vi "Beak Controller.vi"(8 "error in":errorcluster) -> ()   [LabVIEW 2018]
doc: "This VI executes continuously carrying out the current operation and responding to updates or new operations. It will often contain the timing or control code that is difficult to place directly in TeleOp. This VI generally opens all sensors and motors and isolates the rest of the robot code from knowing how the operations are carried out."
uses:
  <vilib>/Rock Robotics/WPI/Framework/Completion Status.ctl
  Beak Setpoints.ctl
  Beak Operations.ctl
  <vilib>/Rock Robotics/WPI/Solenoid/WPI_SolenoidValue.ctl
  <vilib>/Rock Robotics/WPI/Solenoid/WPI_SolenoidDevRef.ctl
  <vilib>/Rock Robotics/WPI/Solenoid/WPI_SolenoidChannel.ctl
  <vilib>/Rock Robotics/WPI/Counter/WPI_CounterDevRef.ctl
  <vilib>/Rock Robotics/SystemInterfaces/Counter/FPGA_CounterCtrSystemIndex.ctl
  <vilib>/Rock Robotics/WPI/Solenoid/WPI_SolenoidSetEnum.vi
  Beak Published Globals.vi
  Wrist/Implementation/Wrist Published Globals.vi
panel:
  in  "Wrist Block Angle":dbl=80.0
  in  "Sensor Distance mm":dbl=60.0
  out "Waveform Chart":dbl(graph)
  out "Distance mm":dbl
  in  "Extend Polarity":T1=enum."Reverse"
  in  "Open Polarity":T1=enum."Reverse"
  in  "Interactive Values":T2
  out "Current\nCmd":string
  in  "Buttons":cluster{"Execute Cmd":bool, "Abort Cmd":bool}
  out "Command Timing":cluster{"Start Time (ms)":u32, "Iterations":i32}
  out "Status":T4
  # "Interactive Command: You may fill in the settings for a command\nand schedule it with the Execute button. You can observe and abort\nany command while fine tuning the code for the controller."
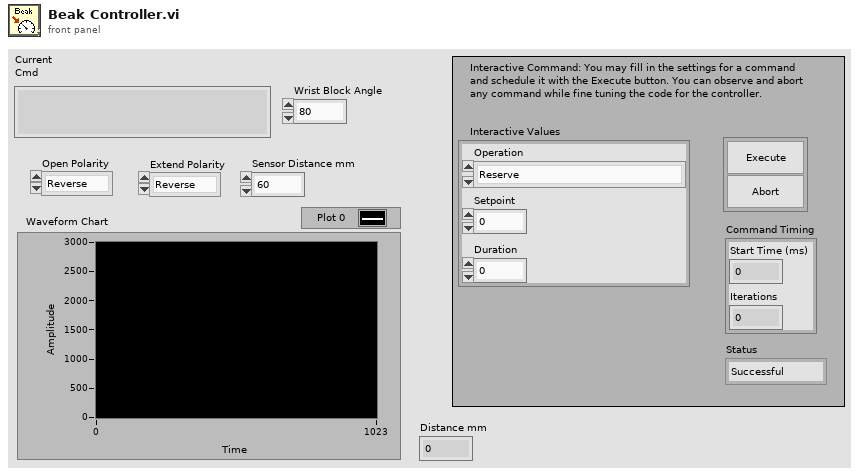
[diagram p1: front panel]
types:
  T1 = typedef "WPI_SolenoidValue.ctl" = enum16{"Off", "On", "Forward", "Reverse"}
  T2 = typedef "Beak Setpoints.ctl" = cluster{"Operation":T3, "Setpoint":dbl, "Duration":dbl}
  T3 = typedef "Beak Operations.ctl" = enum16{"Reserve", "Read Current", "Immediate", "Open", "Close", "Extend", "Retract"}
  T4 = typedef "Completion Status.ctl" = enum16{"Successful", "Aborted", "Incomplete"}
  T5 = typedef "WPI_SolenoidDevRef.ctl" = cluster{"DevStatus":errorcluster, "Pneumatics Control Module":u8, "Forward Solenoid Channel":T6, "Reverse Solenoid Channel":T6}
  T6 = typedef "WPI_SolenoidChannel.ctl" = enum8{"Solenoid 0", "Solenoid 1", "Solenoid 2", "Solenoid 3", "Solenoid 4", "Solenoid 5", "Solenoid 6", "Solenoid 7", "Invalid"}
  T7 = typedef "WPI_CounterDevRef.ctl" = cluster{"DevStatus":errorcluster, "CntIndex":T8}
  T8 = typedef "FPGA_CounterCtrSystemIndex.ctl" = enum8{"Ctr 0", "Ctr 1", "Ctr 2", "Ctr 3", "Ctr 4", "Ctr 5", "Ctr 6", "Ctr 7", "Invalid"}
  T9 = cluster{"Beak":T5, "BeakExtension":T5, "Hatch Sensor":T7}
  T10 = typedef "Command Status Info.ctl" = cluster{"Name":string, "Status":T4, "notifier out":T11}
  T11 = typedef "Completion Notifier.ctl" = refnum<notifier>
  T12 = cluster{"Current Command":T2, "Command Timing":cluster{"Start Time (ms)":u32, "Iterations":i32}, "Command Arguments":cluster{"Command Info":T10, "Description":string, "Default Command":T2, "queue out":refnum<queue>, "Subsystem Name":string}}
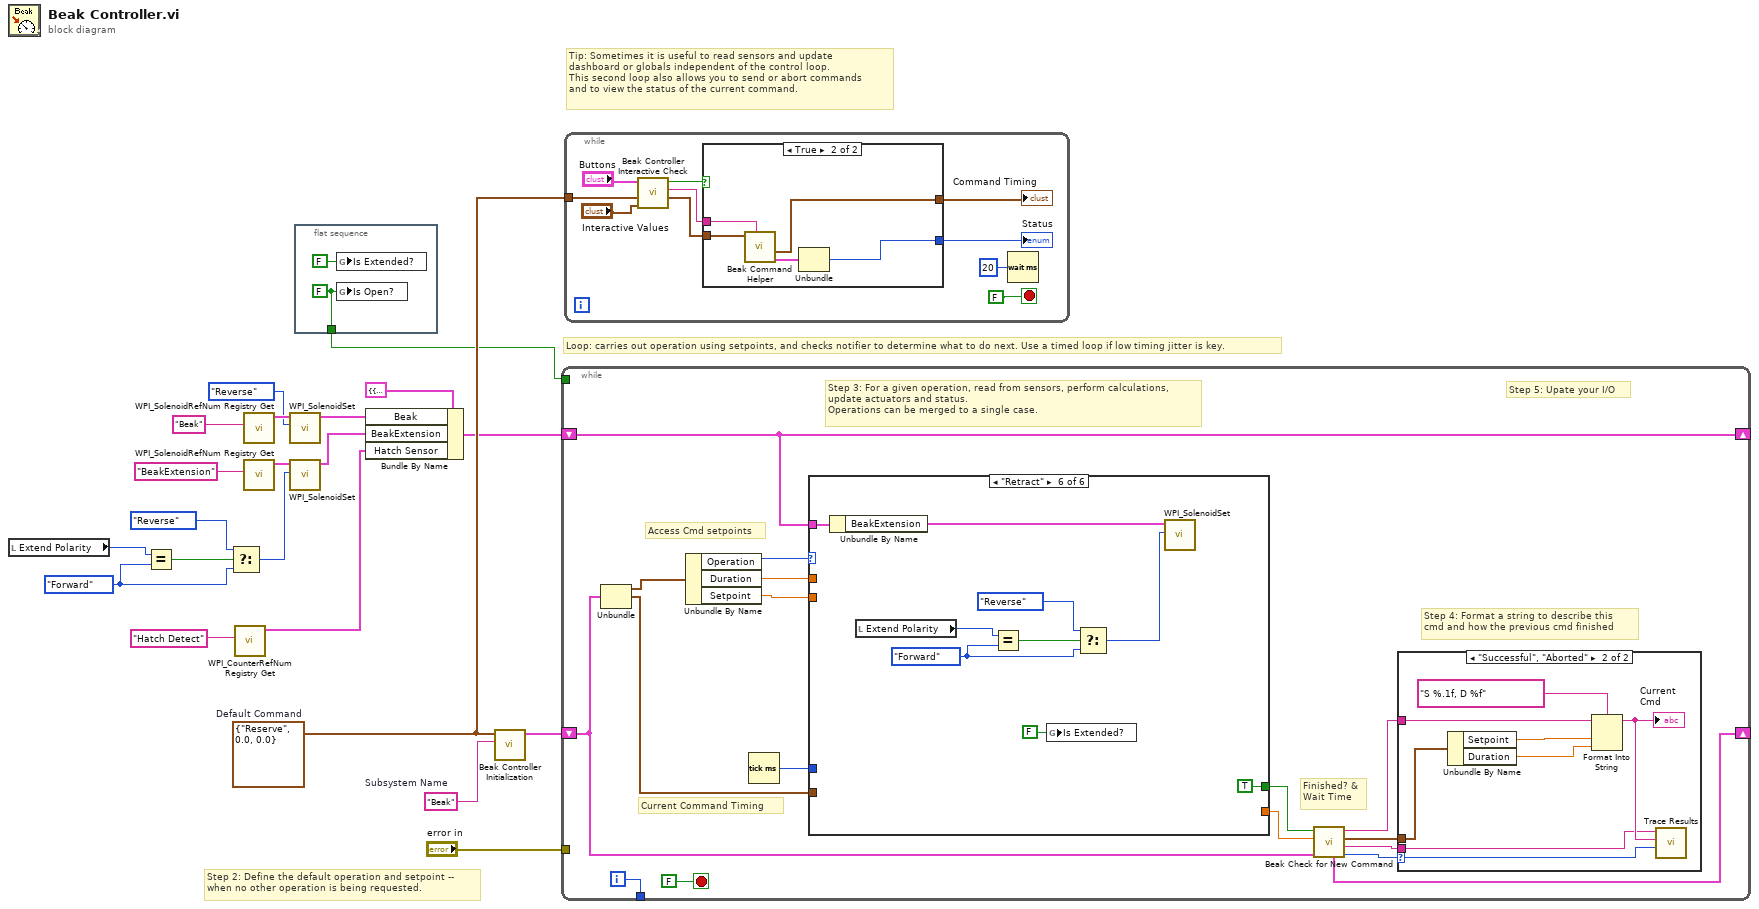
[diagram p0: block diagram]
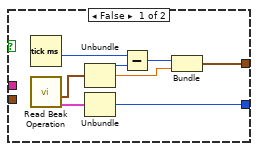
[diagram p2: hidden frame]
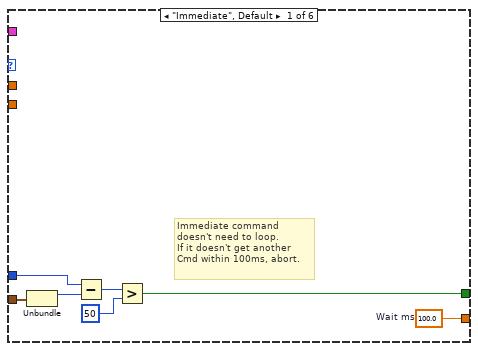
[diagram p4: hidden frame]
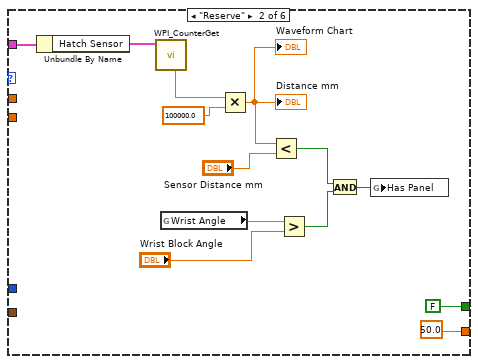
[diagram p5: hidden frame]
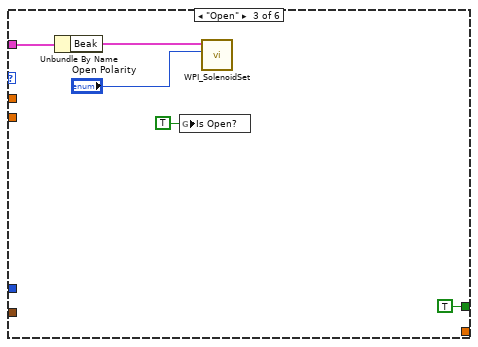
[diagram p6: hidden frame]
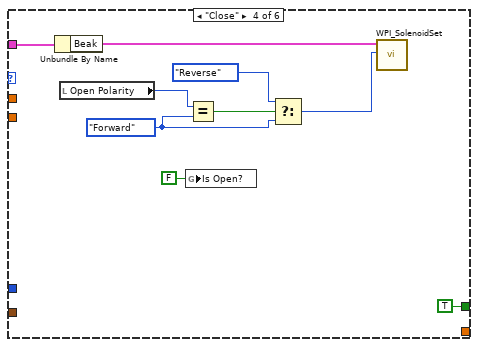
[diagram p7: hidden frame]
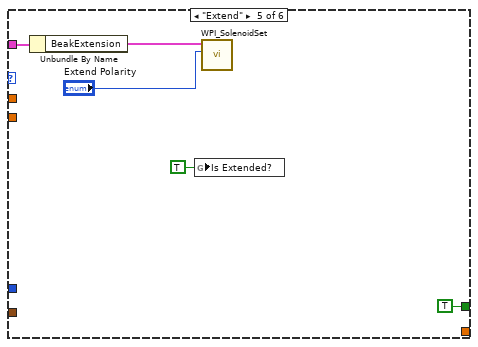
[diagram p8: hidden frame]
diagram:
  w9 = WPI_SolenoidValue."Forward" ("y")
  w18 = T2 {"Operation"=enum."Reserve", "Setpoint"=0.0, "Duration"=0.0}  # Default Command
  w19 = "Beak"  # Subsystem Name
  # "Tip: Sometimes it is useful to read sensors and update\ndashboard or globals independent of the control loop.\nThis second loop also allows you to send or abort commands\nand to view the status of the current command."
  # "Step 2: Define the default operation and setpoint --\nwhen no other operation is being requested."
  # "Loop: carries out operation using setpoints, and checks notifier to determine what to do next. Use a timed loop if low timing jitter is key."
  n1 = local read "Extend Polarity"() -> (w6:T1)
  n2 = Equal?(x=w6, y=w9) -> (x = y?=w7:bool)
  n3 = Select(t=WPI_SolenoidValue."Reverse" ("y"), s=w7, f=w9) -> (s? t:f=w5:T1)
  n4 = call <vilib>:"WPI_CounterRefNum Registry Get.vi"("refnum name"="Hatch Detect") -> ("CounterDevRef"=w3:T7)  [unwired: 9 in, 1 out]
  n5 = call <vilib>:"WPI_SolenoidRefNum Registry Get.vi"("refnum name"="Beak") -> ("SolenoidDevRef"=w13:T5)  [unwired: 9 in, 1 out]
  n6 = call <vilib>:"WPI_SolenoidRefNum Registry Get.vi"("refnum name"="BeakExtension") -> ("SolenoidDevRef"=w11:T5)  [unwired: 9 in, 1 out]
  n7 = call-poly <vilib>:"WPI_SolenoidSet.vi"("Value"=WPI_SolenoidValue."Reverse" ("y"), "SolenoidDevRef"=w13) -> ("SolenoidDevRef"=w12:T5)  [unwired: 8 in, 1 out]
  n8 = call-poly <vilib>:"WPI_SolenoidSet.vi"("Value"=w5, "SolenoidDevRef"=w11) -> ("SolenoidDevRef"=w10:T5)  [unwired: 8 in, 1 out]
  n9 = flat-sequence {
    tunnel: [w22] -> w2
    frame #0 {
      w22 = FALSE ("Is Open?")
      n10 = global write "Beak Published Globals.vi" "Is Extended?"(FALSE ("Is Extended?")) -> ()
      n11 = global write "Beak Published Globals.vi" "Is Open?"(w22) -> ()
    }
  }
  n12 = Bundle By Name(cluster=T9 {"Beak"={"DevStatus"={"status"=FALSE, "code"=0, "source"=""}, "Pneumatics Control Module"=0, "Forward Solenoid Channel"=enum."Invalid", "Reverse Solenoid Channel"=enum."Invalid"}, "BeakExtension"={"DevStatus"={"status"=FALSE, "code"=0, "source"=""}, "Pneumatics Control Module"=0, "Forward Solenoid Channel"=enum."Invalid", "Reverse Solenoid Channel"=enum."Invalid"}, "Hatch Sensor"={"DevStatus"={"status"=FALSE, "code"=0, "source"=""}, "CntIndex"=enum."Ctr 0"}}, "Beak"=w12, "BeakExtension"=w10, "Hatch Sensor"=w3) -> (w14:T9)
  n13 = call "Beak Controller Initialization.vi"("Subsystem Name"=w19, "Default Command"=w18) -> ("Current Command"=w20:T12)  [unwired: 9 in]
  n14 = while {
    shift-right: [w32] -> _
    shift-left: w20 -> [w25]
    tunnel: [w39] -> _
    tunnel: "error in" -> [_]
    shift-right: [w24] -> _
    shift-left: w14 -> [w24]
    tunnel: w2 -> [_]
    i -> [w39]
    stop <- FALSE stop-if-true
    # "Step 5: Upate your I/O"
    # "Step 4: Format a string to describe this\ncmd and how the previous cmd finished"
    # "Current Command Timing"
    # "Access Cmd setpoints"
    # "Finished? &\nWait Time"
    # "Step 3: For a given operation, read from sensors, perform calculations,\nupdate actuators and status.\nOperations can be merged to a single case."
    n15 = Unbundle(w25) -> ("Current Command"=w38:T2, "Command Timing"=w34:cluster{"Start Time (ms)":u32, "Iterations":i32})  [unwired: 1 out]
    n16 = Unbundle By Name(w38) -> ("Operation"=w37:T3, "Duration"=w36:dbl, "Setpoint"=w33:dbl)
    n17 = Tick Count (ms)() -> (millisecond timer value=w35:u32)
    n18 = case shown="\"Retract\"" w37 {
      tunnel: [w55 50.0 _ _ _ _] -> w30
      tunnel: [w49 FALSE ("ignore previous (F)") TRUE ("ignore previous (F)") TRUE ("ignore previous (F)") TRUE ("ignore previous (F)") TRUE ("ignore previous (F)")] -> w31
      tunnel: w34 -> [w51 _ _ _ _ _]
      tunnel: w36 -> [_ _ _ _ _ _]
      tunnel: w35 -> [w50 _ _ _ _ _]
      tunnel: w33 -> [_ _ _ _ _ _]
      tunnel: w24 -> [_ w66 w73 w82 w87 w96]
      frame "Immediate", Default {
        w55 = 100.0  # Wait ms
        # "Immediate command\ndoesn't need to loop.\nIf it doesn't get another\nCmd within 100ms, abort."
        n19 = Unbundle(w51) -> ("Start Time (ms)"=w54:u32)  [unwired: 1 out]
        n20 = Subtract(x=w50, y=w54) -> (x-y=w53:u32)
        n21 = Greater?(x=w53, y=u8 50 ("Left Motor")) -> (0:w49:bool)
      }
      frame "Reserve" {
        n22 = Unbundle By Name(w66) -> ("Hatch Sensor"=w64:T7)
        n23 = call <vilib>:"WPI_CounterGet.vi"("CounterDevRef in"=w64) -> ("Period (sec)"=w63:dbl)  [unwired: 5 in, 5 out]
        n24 = global read "Wrist Published Globals.vi" "Wrist Angle"() -> (w60:dbl)
        n25 = Multiply(x=w63, y=100000.0) -> (x*y=w62:dbl)
        "Distance mm" <- w62
        "Waveform Chart" <- w62
        n26 = Less?(x=w62, y="Sensor Distance mm") -> (x < y?=w58:bool)
        n27 = Greater?(x=w60, y="Wrist Block Angle") -> (0:w57:bool)
        n28 = And(x=w58, y=w57) -> (x .and. y?=w56:bool)
        n29 = global write "Beak Published Globals.vi" "Has Panel"(w56) -> ()
      }
      frame "Open" {
        n30 = Unbundle By Name(w73) -> ("Beak"=w72:T5)
        n31 = global write "Beak Published Globals.vi" "Is Open?"(TRUE ("Is Open?")) -> ()
        n32 = call-poly <vilib>:"WPI_SolenoidSet.vi"("Value"="Open Polarity", "SolenoidDevRef"=w72) -> ()  [unwired: 8 in, 2 out]
      }
      frame "Close" {
        w78 = WPI_SolenoidValue."Forward" ("y")
        n33 = Unbundle By Name(w82) -> ("Beak"=w81:T5)
        n34 = local read "Open Polarity"() -> (w76:T1)
        n35 = global write "Beak Published Globals.vi" "Is Open?"(FALSE ("Is Open?")) -> ()
        n36 = Equal?(x=w76, y=w78) -> (x = y?=w80:bool)
        n37 = Select(t=WPI_SolenoidValue."Reverse" ("y"), s=w80, f=w78) -> (s? t:f=w77:T1)
        n38 = call-poly <vilib>:"WPI_SolenoidSet.vi"("Value"=w77, "SolenoidDevRef"=w81) -> ()  [unwired: 8 in, 2 out]
      }
      frame "Extend" {
        n39 = Unbundle By Name(w87) -> ("BeakExtension"=w86:T5)
        n40 = global write "Beak Published Globals.vi" "Is Extended?"(TRUE ("Is Extended?")) -> ()
        n41 = call-poly <vilib>:"WPI_SolenoidSet.vi"("Value"="Extend Polarity", "SolenoidDevRef"=w86) -> ()  [unwired: 8 in, 2 out]
      }
      frame "Retract" {
        w91 = WPI_SolenoidValue."Forward" ("y")
        n42 = Unbundle By Name(w96) -> ("BeakExtension"=w95:T5)
        n43 = local read "Extend Polarity"() -> (w94:T1)
        n44 = Equal?(x=w94, y=w91) -> (x = y?=w93:bool)
        n45 = global write "Beak Published Globals.vi" "Is Extended?"(FALSE ("Is Extended?")) -> ()
        n46 = Select(t=WPI_SolenoidValue."Reverse" ("y"), s=w93, f=w91) -> (s? t:f=w90:T1)
        n47 = call-poly <vilib>:"WPI_SolenoidSet.vi"("Value"=w90, "SolenoidDevRef"=w95) -> ()  [unwired: 8 in, 2 out]
      }
    }
    n48 = call "Beak Check for New Command.vi"("Current Command"=w25, "Wait time (ms)"=w30, "Finished?"=w31) -> ("Completion"=w26:T4, "Subsystem Name"=w27:string, "Current Command"=w28:T2, "Initial Trace String"=w29:string, "NextCommand"=w32:T12)  [unwired: 4 in]
    n49 = case shown="\"Successful\", \"Aborted\"" w26 {
      selector: w26 -> [_ w48]
      tunnel: w29 -> [_ w44]
      tunnel: w28 -> [_ w45]
      tunnel: w27 -> [_ w41]
      frame "Incomplete", Default {
        # "Continuing current command"
      }
      frame "Successful", "Aborted" {
        # "Report and setup for next command"
        n50 = Unbundle By Name(w45) -> ("Setpoint"=w47:dbl, "Duration"=w42:dbl)
        n51 = Format Into String(format string="S %.1f, D %f", initial string=w44, w47, w42) -> (resulting string=w43:string)  [unwired: 1 in, 1 out]
        "Current\nCmd" <- w43
        n52 = call <vilib>:"Trace Results.vi"("Status of previous command"=w48, "Description"=w43, "Subsystem"=w41) -> ()  [unwired: 9 in]
      }
    }
  }
  n53 = while {
    tunnel: w18 -> [w103]
    stop <- FALSE stop-if-true
    n54 = call "Beak Controller Interactive Check.vi"("Interactive Command in"="Interactive Values", "Default Command"=w103, "Buttons"="Buttons") -> ("Interactive Command out"=w100:T2, "Trace String"=w101:string, "Schedule"=w102:bool)  [unwired: 6 in]
    n55 = case shown="True" w102 {
      tunnel: [w114 w119] -> w99
      tunnel: w100 -> [_ w117]
      tunnel: [w110 w115] -> w98
      tunnel: w101 -> [_ w118]
      frame False {
        n56 = Tick Count (ms)() -> (millisecond timer value=w109:u32)
        n57 = call "Read Beak Operation.vi"() -> ("Command Info"=w107:T10, "SubSystem Data"=w108:T2)  [unwired: 9 in, 1 out]
        n58 = Unbundle(w108) -> ("Operation"=w113:T3, "Setpoint"=w111:dbl)  [unwired: 1 out]
        n59 = Unbundle(w107) -> ("Status"=w114:T4)  [unwired: 2 out]
        n60 = Subtract(x=w109, y=w113) -> (x-y=w112:u32)
        n61 = Bundle(w112, "Setpoint"=w111) -> (w110:cluster{u32, "Setpoint":dbl})  [unwired: 1 in]
      }
      frame True {
        n62 = call "Beak Command Helper.vi"("Description"=w118, "SubSystem Data"=w117) -> ("Command Info Out"=w116:T10, "Command Timing"=w115:cluster{"Start Time (ms)":u32, "Iterations":i32})  [unwired: 7 in, 1 out]
        n63 = Unbundle(w116) -> ("Status"=w119:T4)  [unwired: 2 out]
      }
    }
    "Status" <- w99
    "Command Timing" <- w98
    n64 = Wait (ms)(milliseconds to wait=u32 20) -> ()  [unwired: 1 out]
  }
